vi "QPSK - Copy.vi"(8 "ebn0":dbl=4.0) -> (0 "Pr(error) ideal":dbl=0.012500818040737566, 1 "Pr(error) measured":dbl=0.012500818040737566, 2 "Histogram (cos)":dynamicdata(graph)=[{"t0"=timestamp(-1.485 s since 1904-01-01), "dt"=0.03, "Y"=[0.0, 0.0, 0.0, 0.0, 0.0, 0.0, 0.0, 0.0, 0.0, 0.0, 0.0, 0.0, 0.0, 0.0, 0.0, 0.0, 0.0, 0.0, 0.0, 0.0, 0.0, 0.0, 0.0, 0.0, 0.0, 0.0, 0.0, 0.0, 0.0, 0.0, 0.0, 0.0, 0.0, 0.0, 0.0, 0.0, 0.0, 0.0, 0.0, 0.0, 0.0, 0.0, 0.0, 0.0, 0.0, 0.3, 0.2, 0.0, 0.5, 0.4, 0.4, 0.6, 1.0999999999999999, 1.3, 1.5, 1.2, 2.5, 2.9000000000000004, 2.8000000000000003, 3.4000000000000004, 5.0, 4.3, 4.1000000000000005, 3.5999999999999996, 4.6, 5.3, 5.4, 6.0, 5.5, 5.4, 5.4, 4.3, 3.5999999999999996, 3.5000000000000004, 2.3, 3.0, 1.7000000000000002, 1.4000000000000001, 1.5, 0.7000000000000001, 1.5, 0.6, 0.5, 0.4, 0.6, 0.1, 0.2, 0.1, 0.2, 0.1, 0.0, 0.0, 0.0, 0.0, 0.0, 0.0, 0.0, 0.0, 0.0, 0.0], "attributes"=variant("NI_ChannelName"=variant(string " (Histogram)"), "NI_ExpIsRelativeTime"=variant(bool TRUE), "NI_ExpStartTimeStamp"=variant(timestamp timestamp(3729531312.5421457 s since 1904-01-01)), "NI_ExpTimeStamp"=variant(timestamp timestamp(3729531312.5421457 s since 1904-01-01)), "NI_ExpXDimension"=variant(string "BIN"), "NI_OriginalChannelName"=variant(string ""))}] caption="Histogram", 3 "Histogram (sin)":dynamicdata(graph)=[{"t0"=timestamp(-1.485 s since 1904-01-01), "dt"=0.03, "Y"=[0.0, 0.0, 0.0, 0.0, 0.0, 0.0, 0.0, 0.0, 0.0, 0.0, 0.0, 0.0, 0.0, 0.0, 0.0, 0.0, 0.0, 0.0, 0.0, 0.0, 0.0, 0.0, 0.0, 0.0, 0.0, 0.0, 0.0, 0.0, 0.0, 0.0, 0.0, 0.0, 0.0, 0.0, 0.0, 0.0, 0.0, 0.0, 0.0, 0.0, 0.0, 0.0, 0.0, 0.0, 0.0, 0.1, 0.2, 0.1, 0.3, 0.3, 0.1, 0.7000000000000001, 0.6, 0.8, 1.2, 1.2, 2.9000000000000004, 1.7999999999999998, 2.8000000000000003, 5.3, 3.9, 5.5, 4.0, 4.3999999999999995, 5.1, 3.8, 4.7, 5.3, 4.8, 4.5, 3.9, 5.1, 4.3, 3.9, 3.8, 3.1, 2.9000000000000004, 1.3, 1.7999999999999998, 0.8, 1.0999999999999999, 0.6, 0.8, 0.7000000000000001, 0.6, 0.6, 0.2, 0.1, 0.0, 0.0, 0.0, 0.0, 0.0, 0.0, 0.0, 0.0, 0.0, 0.0, 0.0, 0.0], "attributes"=variant("NI_ChannelName"=variant(string " (Histogram)"), "NI_ExpIsRelativeTime"=variant(bool TRUE), "NI_ExpStartTimeStamp"=variant(timestamp timestamp(3729531312.5421457 s since 1904-01-01)), "NI_ExpTimeStamp"=variant(timestamp timestamp(3729531312.5421457 s since 1904-01-01)), "NI_ExpXDimension"=variant(string "BIN"), "NI_OriginalChannelName"=variant(string ""))}] caption="Histogram", 6 "Sigma_out (measured)":dbl format="%.6f", 7 "Sigma_out (Ideal)":dbl)   [LabVIEW 2019]
uses:
  <vilib>/imath/engines/lvmath2/RunTimeEngine/NodeEndStatement/NIMS_NodeEndStatement_Output.vi
  <instcachedir>/0/NIMS_NodeEndStatement_Output_53EC0D466D134D7ABD903AC30B43404B.lvgen/NIMS_NodeEndStatement_Output_53EC0D466D134D7ABD903AC30B43404B_009.vi
  <vilib>/imath/engines/lvmath2/RunTimeEngine/ErrorHandling/NIMS_Finalize Error.vi
  <vilib>/measure/NI_MABase.lvlib
  <vilib>/gmath/NI_Gmath.lvlib
  <vilib>/Analysis/NI_AALBase.lvlib
panel:
  out "Graphs (sin)":waveform(dbl)[](graph)=[{"t0"=timestamp(0 s since 1904-01-01), "dt"=0.01, "Y"=array[1000 elements]}, {"t0"=timestamp(0 s since 1904-01-01), "dt"=0.01, "Y"=array[1000 elements]}, {"t0"=timestamp(0 s since 1904-01-01), "dt"=0.01, "Y"=array[1000 elements]}, {"t0"=timestamp(0 s since 1904-01-01), "dt"=0.01, "Y"=array[1000 elements], "attributes"=variant("NI_ChannelName"=variant(string "Integral (Sum[Xdt])"))}, {"t0"=timestamp(0 s since 1904-01-01), "dt"=0.01, "Y"=array[1000 elements], "attributes"=variant("NI_ChannelName"=variant(string "Integral (Sum[Xdt])"))}]
  out "I_out (sin)":dbl=0.5375925976458646
  out "s(t) amplitude":dbl=0.10023744672545445
  in  "s":dbl=1000.0
  in  "sigma_in 2":dbl=1.0
  out "T":dbl=10.0
  out "E_b":dbl=0.050237728630191596
  out "E_b / N_0 (dB)":dbl=3.999999999999999
  out "E_b / N_0":dbl=2.5118864315095797
  out "N_0":dbl=0.02
  in  "sampling info":cluster{"Fs":dbl, "#s":dbl}={"Fs"=100.0, "#s"=1000.0} {"Fs" format="%.2p"}
  out "Graphs (cos)":waveform(dbl)[](graph)=[{"t0"=timestamp(0 s since 1904-01-01), "dt"=0.01, "Y"=array[1000 elements]}, {"t0"=timestamp(0 s since 1904-01-01), "dt"=0.01, "Y"=array[1000 elements]}, {"t0"=timestamp(0 s since 1904-01-01), "dt"=0.01, "Y"=array[1000 elements]}, {"t0"=timestamp(0 s since 1904-01-01), "dt"=0.01, "Y"=array[1000 elements], "attributes"=variant("NI_ChannelName"=variant(string "Integral (Sum[Xdt])"))}, {"t0"=timestamp(0 s since 1904-01-01), "dt"=0.01, "Y"=array[1000 elements], "attributes"=variant("NI_ChannelName"=variant(string "Integral (Sum[Xdt])"))}]
  out "I_out (cos)":dbl=0.13330337863726935
  in  "oscillator frequency":dbl=1.0 format="%0.2p"
  in  "oscillator amplitude":dbl=1.0 format="%0.2p"
  in  "s(t) frequency":dbl=1.0 format="%0.2p"
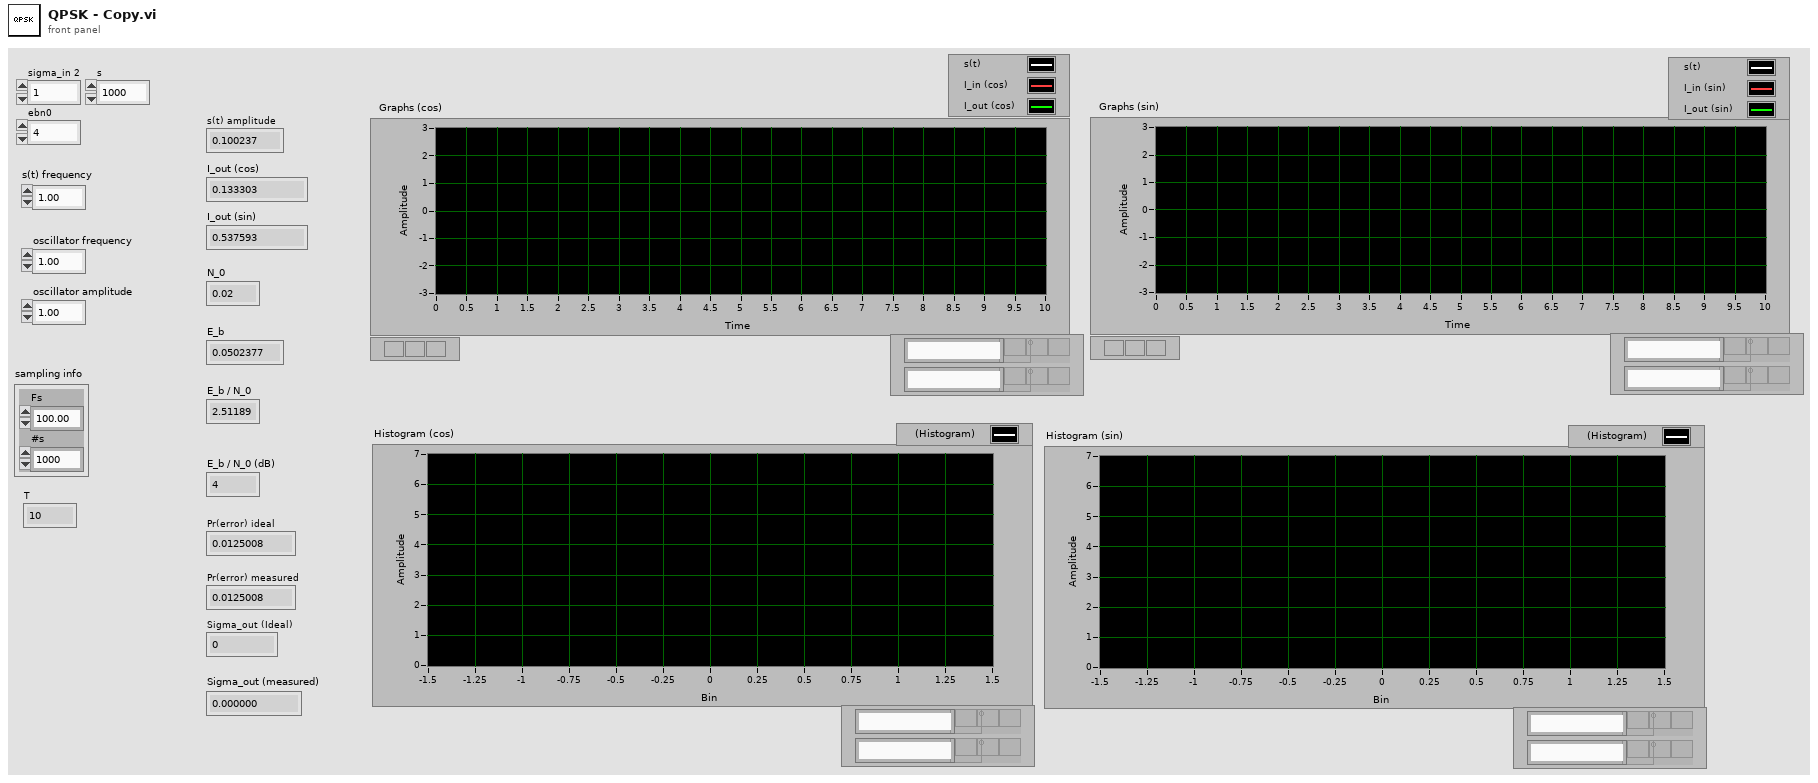
[diagram p1: front panel]
types:
  T1 = enum16{"Sine Wave", "Triangle Wave", "Square Wave", "Sawtooth Wave"}
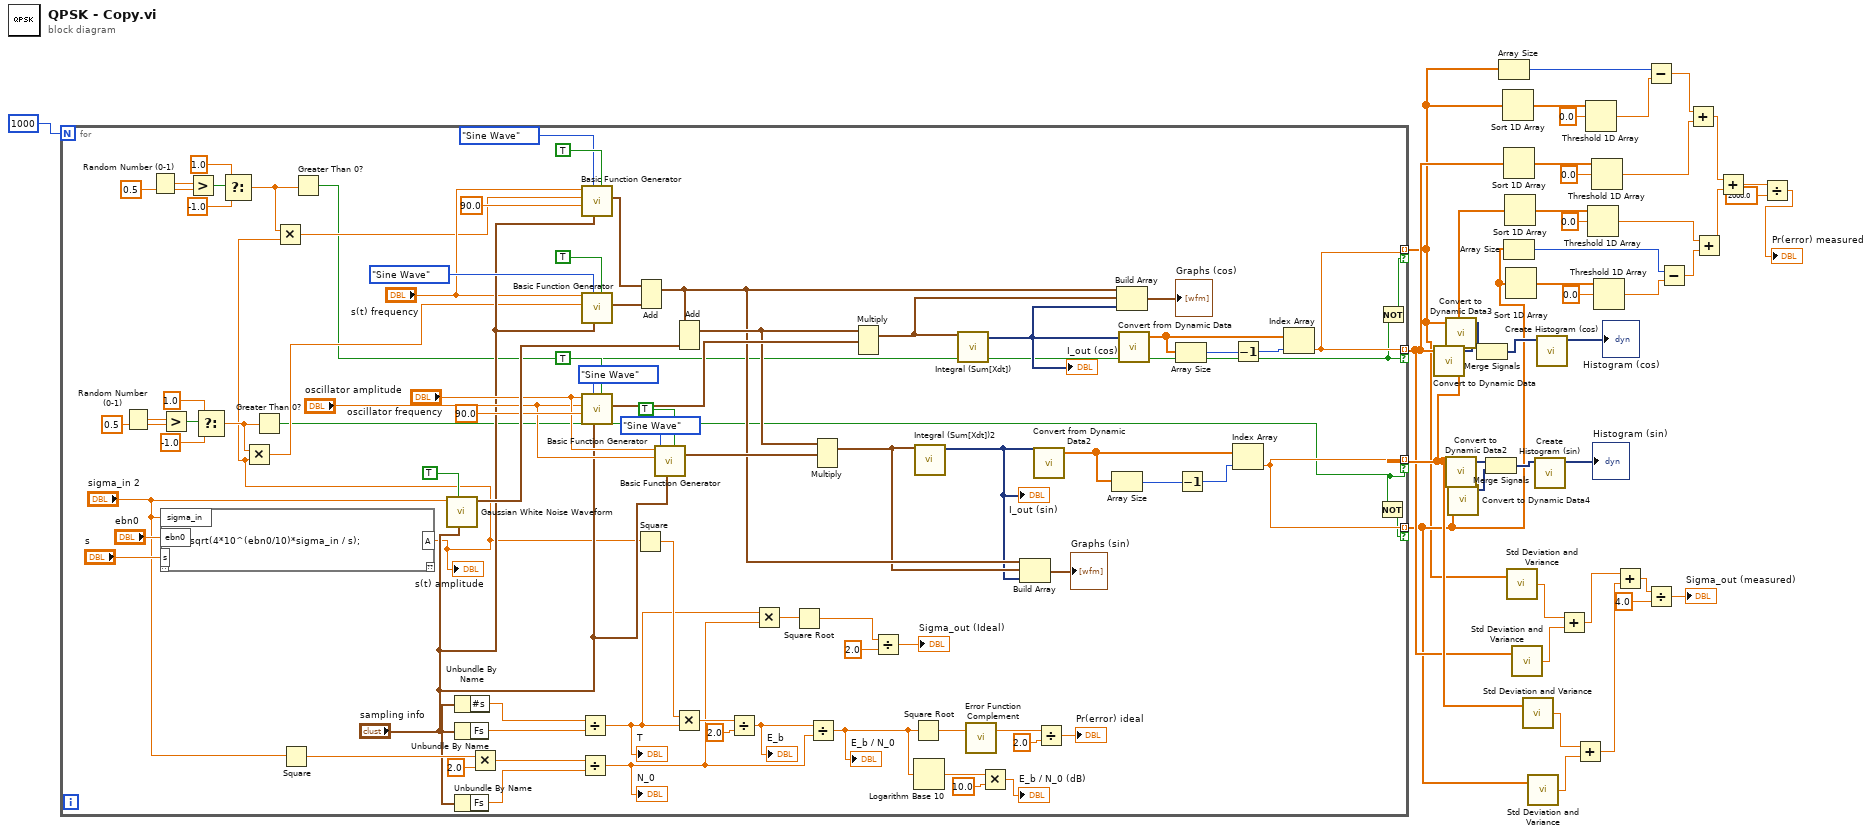
[diagram p0: block diagram]
diagram:
  n1 = for {
    N: 1000 -> [_]
    tunnel: [w53] -> w10 mode=indexing if=w52
    tunnel: [w56] -> w17 mode=indexing if=w55
    tunnel: [w56] -> w8 mode=indexing if=w54
    tunnel: [w53] -> w4 mode=indexing if=w51
    n2 = Random Number (0-1)() -> (number: 0 to 1=w73:dbl)
    n3 = Random Number (0-1)() -> (number: 0 to 1=w77:dbl)
    n4 = Greater?(x=w73, y=0.5) -> (0:w72:bool)
    n5 = mathscript code="A = sqrt(4*10^(ebn0/10)*sigma_in / s);"("s"="s", "ebn0"="ebn0", "sigma_in"="sigma_in 2") -> ("A"=w45:cdb)  [unwired: 1 in, 1 out]
    "s(t) amplitude" <- w45
    n6 = Greater?(x=w77, y=0.5) -> (0:w76:bool)
    n7 = Select(t=1.0, s=w72, f=-1.0) -> (s? t:f=w59:dbl)
    n8 = Select(t=1.0, s=w76, f=-1.0) -> (s? t:f=w60:dbl)
    n9 = Multiply(x=w59, y=w45) -> (x*y=w58:cdb)
    n10 = Greater Than 0?(x=w59) -> (x > 0?=w55:bool)
    n11 = Multiply(x=w60, y=w45) -> (x*y=w57:cdb)
    n12 = Square(x="sigma_in 2") -> (x^2=w113:dbl)
    n13 = Greater Than 0?(x=w60) -> (x > 0?=w52:bool)
    n14 = call <vilib>:"Gaussian White Noise Waveform.vi"("sampling info"="sampling info", "reset signal"=TRUE, "standard deviation"="sigma_in 2") -> ("signal out"=w111:waveform(dbl))  [unwired: 7 in, 1 out]
    n15 = Unbundle By Name("sampling info") -> ("#s"=w94:dbl)
    n16 = Unbundle By Name("sampling info") -> ("Fs"=w122:dbl)
    n17 = Unbundle By Name("sampling info") -> ("Fs"=w115:dbl)
    n18 = Multiply(x=w113, y=2.0) -> (x*y=w114:dbl)
    n19 = Divide(x=w94, y=w122) -> (x/y=w44:dbl)
    "T" <- w44
    n20 = Divide(x=w114, y=w115) -> (x/y=w46:dbl)
    "N_0" <- w46
    n21 = call <vilib>:"Basic Function Generator.vi"("reset signal"=TRUE, "sampling info"="sampling info", "signal type"=T1."Sine Wave", "phase"=90.0, "amplitude"=w57, "frequency"="s(t) frequency") -> ("signal out"=w109:waveform(dbl))  [unwired: 3 in, 2 out]
    n22 = call <vilib>:"Basic Function Generator.vi"("reset signal"=TRUE, "sampling info"="sampling info", "signal type"=T1."Sine Wave", "amplitude"=w58, "frequency"="s(t) frequency") -> ("signal out"=w110:waveform(dbl))  [unwired: 4 in, 2 out]
    n23 = call <vilib>:"Basic Function Generator.vi"("reset signal"=TRUE, "sampling info"="sampling info", "signal type"=T1."Sine Wave", "phase"=90.0, "amplitude"="oscillator amplitude", "frequency"="oscillator frequency") -> ("signal out"=w112:waveform(dbl))  [unwired: 3 in, 2 out]
    n24 = Square(x=w45) -> (x^2=w117:cdb)
    n25 = Add(1:w110, 2:w109) -> (0:w67:waveform(dbl))  [unwired: 1 in, 1 out]
    n26 = call <vilib>:"Basic Function Generator.vi"("reset signal"=TRUE, "sampling info"="sampling info", "signal type"=T1."Sine Wave" ("oscillator (sin)"), "amplitude"="oscillator amplitude", "frequency"="oscillator frequency") -> ("signal out"=w84:waveform(dbl))  [unwired: 4 in, 2 out]
    n27 = Add(1:w111, 2:w67) -> (0:w85:waveform(dbl))  [unwired: 1 in, 1 out]
    n28 = Multiply(x=w117, y=w44) -> (x*y=w118:cdb)
    n29 = Divide(x=w118, y=2.0) -> (x/y=w119:cdb)
    "E_b" <- w119
    n30 = Multiply(x=w44, y=w46) -> (x*y=w50:dbl)
    n31 = Square Root(x=w50) -> (sqrt(x)=w48:dbl)
    n32 = Divide(x=w119, y=w46) -> (x/y=w89:cdb)
    "E_b / N_0" <- w89
    n33 = Multiply(1:w84, 2:w85) -> (0:w66:waveform(dbl))  [unwired: 1 in, 1 out]
    n34 = Multiply(1:w112, 2:w85) -> (0:w120:waveform(dbl))  [unwired: 1 in, 1 out]
    n35 = Divide(x=w48, y=2.0) -> (x/y=→"Sigma_out (Ideal)":dbl)
    n36 = Square Root(x=w89) -> (sqrt(x)=w97:cdb)
    n37 = Logarithm Base 10(1:w89) -> (0:w116:cdb)
    n38 = call "Integral (Sum[Xdt])2"("Signals"=w66) -> ("Result"=w65:dynamicdata)  [unwired: 5 in, 1 out]
    "I_out (sin)" <- w65
    n39 = call "Integral (Sum[Xdt])"("Signals"=w120) -> ("Result"=w69:dynamicdata)  [unwired: 5 in, 1 out]
    "I_out (cos)" <- w69
    n40 = call <vilib>:"Error Function Complement.vi"("x"=w97) -> ("1 - erf(x)"=w96:dbl)  [unwired: 2 in]
    n41 = Multiply(x=w116, y=10.0) -> (x*y=→"E_b / N_0 (dB)":cdb)
    n42 = Build Array(w67, w66, w65) -> (→"Graphs (sin)":waveform(dbl)[])
    n43 = call "Convert from Dynamic Data2"("Dynamic Data Type"=w65) -> ("Array"=w80:dbl[])  [unwired: 3 in]
    n44 = Divide(x=w96, y=2.0) -> (x/y=→"Pr(error) ideal":dbl)
    n45 = Array Size(array=w80) -> (size(s)=w79:i32)
    n46 = Build Array(w67, w120, w69) -> (→"Graphs (cos)":waveform(dbl)[])
    n47 = call "Convert from Dynamic Data"("Dynamic Data Type"=w69) -> ("Array"=w123:dbl[])  [unwired: 3 in]
    n48 = Array Size(array=w123) -> (size(s)=w124:i32)
    n49 = Decrement(x=w79) -> (x-1=w78:i32)
    n50 = Decrement(x=w124) -> (x-1=w125:i32)
    n51 = Index Array(array=w80, index=w78) -> (element=w56:dbl)
    n52 = Index Array(array=w123, index=w125) -> (element=w53:dbl)
    n53 = Not(x=w55) -> (.not. x?=w54:bool)
    n54 = Not(x=w52) -> (.not. x?=w51:bool)
  }
  n55 = call "Convert to Dynamic Data"("Array"=w10) -> ("Dynamic Data Type"=w41:dynamicdata)  [unwired: 3 in]
  n56 = call "Convert to Dynamic Data3"("Array"=w4) -> ("Dynamic Data Type"=w37:dynamicdata)  [unwired: 3 in]
  n57 = call "Convert to Dynamic Data2"("Array"=w17) -> ("Dynamic Data Type"=w40:dynamicdata)  [unwired: 3 in]
  n58 = call "Convert to Dynamic Data4"("Array"=w8) -> ("Dynamic Data Type"=w35:dynamicdata)  [unwired: 3 in]
  n59 = Merge Signals(w41, w37) -> (w38:dynamicdata)
  n60 = Merge Signals(w40, w35) -> (w36:dynamicdata)
  n61 = Array Size(array=w4) -> (size(s)=w9:i32)
  n62 = Sort 1D Array(array=w4) -> (sorted array=w25:dbl[])
  n63 = Sort 1D Array(array=w10) -> (sorted array=w23:dbl[])
  n64 = Array Size(array=w8) -> (size(s)=w6:i32)
  n65 = Sort 1D Array(array=w17) -> (sorted array=w21:dbl[])
  n66 = Sort 1D Array(array=w8) -> (sorted array=w19:dbl[])
  n67 = call <vilib>:"Std Deviation and Variance.vi"("X"=w4) -> ("standard deviation"=w34:dbl)  [unwired: 1 in, 2 out]
  n68 = call <vilib>:"Std Deviation and Variance.vi"("X"=w10) -> ("standard deviation"=w33:dbl)  [unwired: 1 in, 2 out]
  n69 = call <vilib>:"Std Deviation and Variance.vi"("X"=w17) -> ("standard deviation"=w31:dbl)  [unwired: 1 in, 2 out]
  n70 = call <vilib>:"Std Deviation and Variance.vi"("X"=w8) -> ("standard deviation"=w30:dbl)  [unwired: 1 in, 2 out]
  n71 = call "Create Histogram (sin)"("Signal"=w36) -> ("Histogram"=→"Histogram (sin)":dynamicdata)  [unwired: 9 in, 1 out]
  n72 = call "Create Histogram (cos)"("Signal"=w38) -> ("Histogram"=→"Histogram (cos)":dynamicdata)  [unwired: 9 in, 1 out]
  n73 = Add(x=w34, y=w33) -> (x+y=w29:dbl)
  n74 = Add(x=w31, y=w30) -> (x+y=w28:dbl)
  n75 = Threshold 1D Array(2:0.0 ("threshold y"), 3:w25) -> (0:w3:dbl)  [unwired: 1 in]
  n76 = Threshold 1D Array(2:0.0 ("threshold y"), 3:w21) -> (0:w7:dbl)  [unwired: 1 in]
  n77 = Threshold 1D Array(2:0.0 ("threshold y"), 3:w23) -> (0:w1:dbl)  [unwired: 1 in]
  n78 = Threshold 1D Array(2:0.0 ("threshold y"), 3:w19) -> (0:w5:dbl)  [unwired: 1 in]
  n79 = Add(x=w29, y=w28) -> (x+y=w27:dbl)
  n80 = Subtract(x=w9, y=w3) -> (x-y=w2:dbl)
  n81 = Divide(x=w27, y=4.0) -> (x/y=→"Sigma_out (measured)":dbl)
  n82 = Subtract(x=w6, y=w5) -> (x-y=w11:dbl)
  n83 = Add(x=w2, y=w1) -> (x+y=w15:dbl)
  n84 = Add(x=w7, y=w11) -> (x+y=w16:dbl)
  n85 = Add(x=w15, y=w16) -> (x+y=w14:dbl)
  n86 = Divide(x=w14, y=2000.0) -> (x/y=→"Pr(error) measured":dbl)
